vi "OCR_Characterize Rows.vi"(7 "Frame":T2, 8 "Error":errorcluster, 11 "2D Image":T3) -> (0 "Error Out":errorcluster, 2 "Top Color Array Out":T1[](array[typedef]), 3 "Row Type Out":T4[](array[typedef]))   [LabVIEW 2009]
doc: "Characterizes each Row in the 2D color image."
uses:
  Controls/Enum/ENUM_Line Letter Type.ctl
  Controls/Array/Color Box Array_2D Icon Viewer.ctl
  Controls/Enum/ENUM_Frame Template Select.ctl
  Controls/Cluster/Cluster_Text Color Set.ctl
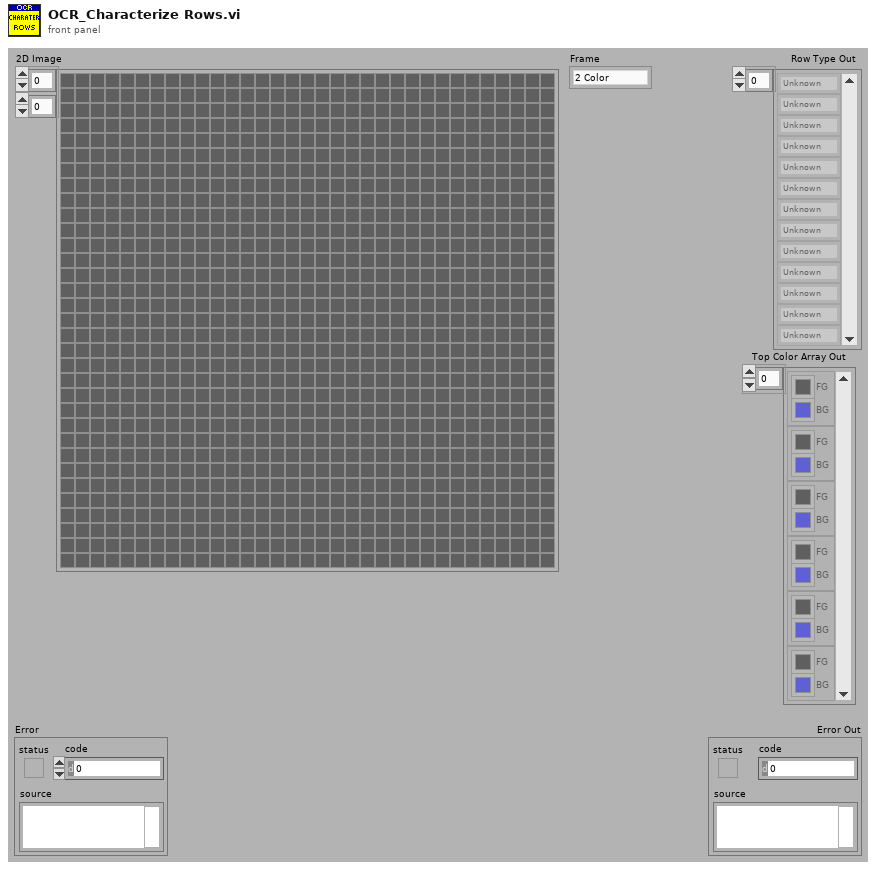
[diagram p1: front panel]
types:
  T1 = typedef "Cluster_Text Color Set.ctl" = cluster{"BG":u32, "FG":u32}
  T2 = typedef "ENUM_Frame Template Select.ctl" = enum16{"2 Color", "5 Color"}
  T3 = typedef "Color Box Array_2D Icon Viewer.ctl" = u32[][]
  T4 = typedef "ENUM_Line Letter Type.ctl" = enum16{"Unknown", "Letter", "Seperator", "Seperator or Letter"}
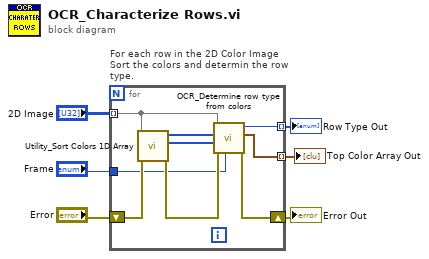
[diagram p0: block diagram]
diagram:
  n1 = for "For each row in the 2D Color Image\nSort the colors and determin the row\ntype." {
    tunnel: "2D Image" -> [w8] mode=indexing
    tunnel: [w10] -> w6 mode=indexing
    shift-right: [w13] -> w4
    shift-left: "Error" -> [w15]
    tunnel: "Frame" -> [w9]
    tunnel: [w7] -> w1 mode=indexing
    n2 = call "Utility_Sort Colors 1D Array.vi"("Error"=w15, "Colors"=w8) -> ("Error Out"=w14:errorcluster, "Count Out"=w11:u32[], "Sorted By Quantity Out"=w12:u32[])  [unwired: 7 in]
    n3 = call "OCR_Determine row type from colors.vi"("Frame"=w9, "Error"=w14, "Count"=w11, "Sorted By Quantity"=w12, "Color List"=w8) -> ("Error Out"=w13:errorcluster, "Highest Quanity Colors Out"=w7:T1, "Type Out"=w10:T4)  [unwired: 4 in]
  }
  "Row Type Out" <- w6
  "Error Out" <- w4
  "Top Color Array Out" <- w1
